vi "LDC501Control.vi"() -> ()   [LabVIEW 2021]
uses:
  <vilib>/Utility/file.llb/Write Delimited Spreadsheet (DBL).vi
panel:
  in  "LASER CONFIGURATION 2":T1={"LD Range"=1, "Laser Control Mode"=0, "Laser Mod On/OFF"=1, "Laser Mod BW"=1} {"Laser Mod BW" items=["Low", "High"]; "Laser Mod On/OFF" items=["OFF", "ON"]; "Laser Control Mode" items=["CC", "CP"]; "LD Range" items=["250mA", "500mA"]}
  in  "LASER CONFIGURATION":T1={"LD Range"=1, "Laser Control Mode"=0, "Laser Mod On/OFF"=1, "Laser Mod BW"=1} {"Laser Mod BW" items=["Low", "High"]; "Laser Mod On/OFF" items=["OFF", "ON"]; "Laser Control Mode" items=["CC", "CP"]; "LD Range" items=["250mA", "500mA"]}
  in  "LASER LIMIT & TRIP-OFF 2":T2
  in  "LASER LIMIT & TRIP-OFF":T2
  out "Laser On 2":bool
  out "LD Voltage":dbl
  out "LD Current":dbl
  in  "Laser ON/OFF 2":bool
  in  "LD Setting Point":dbl
  in  "Repump Laser":refnum<visa-resource-name>="LDC_Repump"
  out "error out 2":errorcluster
  out "error out":errorcluster
  out "LD Voltage":dbl
  out "LD Current":dbl
  in  "LD Setting Point":dbl
  out "Laser On":bool
  in  "Laser ON/OFF":bool
  in  "Refresh Monitor":bool
  in  "Trap Laser":refnum<visa-resource-name>="LDC_Trap"
  in  "Stop":bool
  in  "Export Setting":bool
  in  "Import Setting":bool
  # "Trap & Repump Laser Controller"
  # "LD Currernt Range"
  # "Laser Control Mode"
  # "Laser Mod On/OFF"
  # "Laser Mod BW"
  # "LD Currernt Range"
  # "Laser Control Mode"
  # "Laser Mod On/OFF"
  # "Laser Mod BW"
  # "Laser Trip-off on"
  # "Current Limit"
  # "TEC Off"
  # "Min Temperature"
  # "Max Temperature"
  # "Laser Trip-off on"
  # "Current Limit"
  # "TEC Off"
  # "Min Temperature"
  # "Max Temperature"
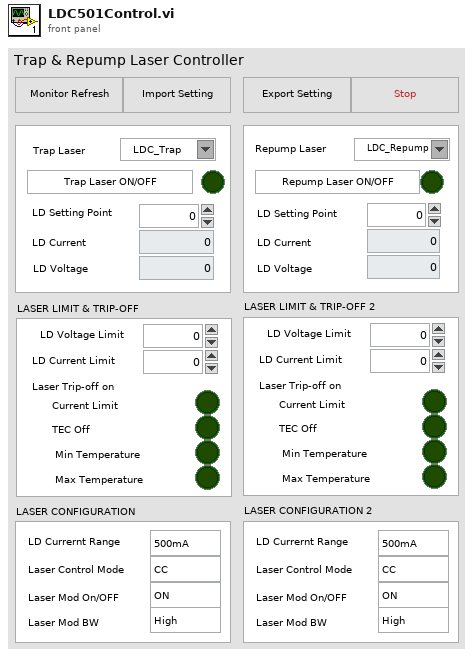
[diagram p1: front panel]
types:
  T1 = cluster{"LD Range":u16, "Laser Control Mode":u16, "Laser Mod On/OFF":u16, "Laser Mod BW":u16}
  T2 = cluster{"LD Voltage Limit":dbl, "LD Current Limit":dbl, "Laser Trip-off on Current Limit":bool, "Laser Trip-off on TEC Off":bool, "Laser Trip-off on Min Temperature":bool, "Laser Trip-off on Max Temperature":bool}
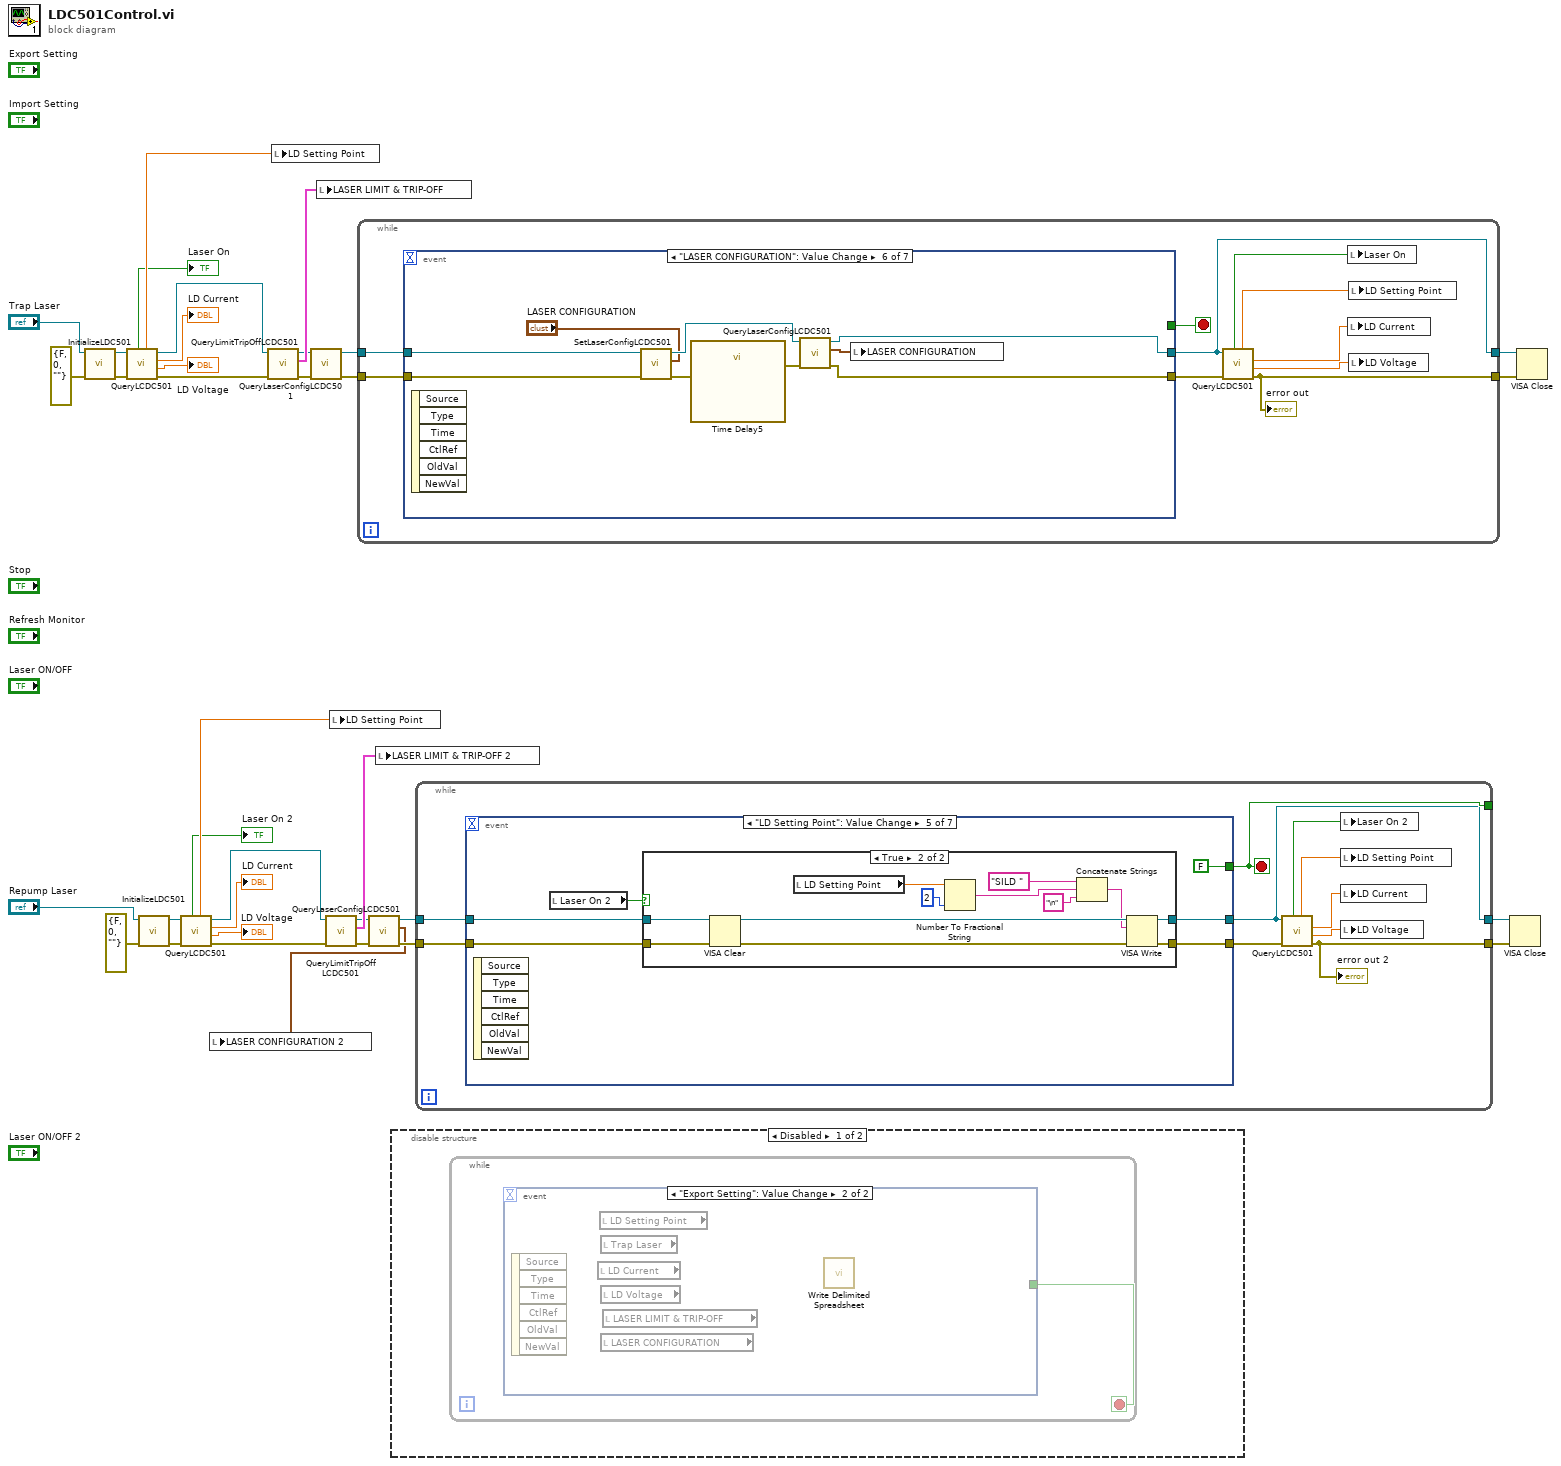
[diagram p0: block diagram]
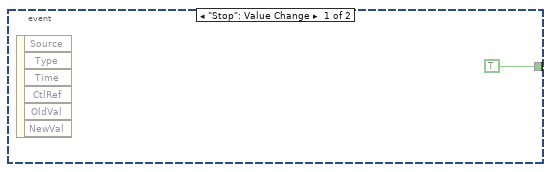
[diagram p2: hidden frame]
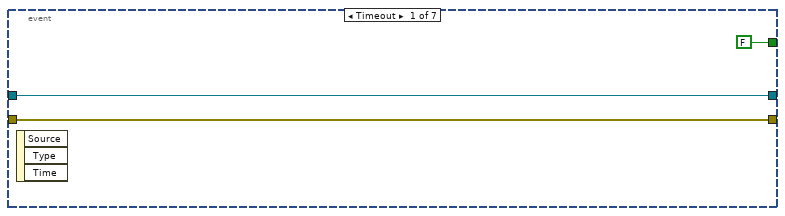
[diagram p4: hidden frame]
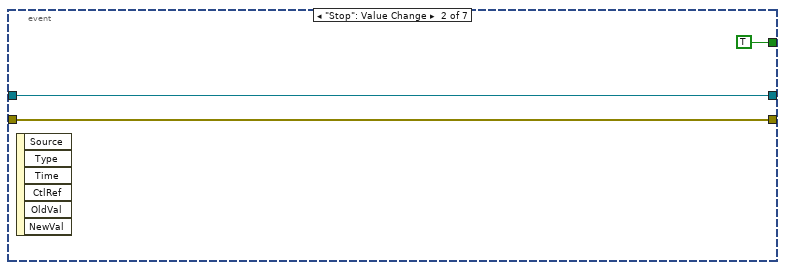
[diagram p5: hidden frame]
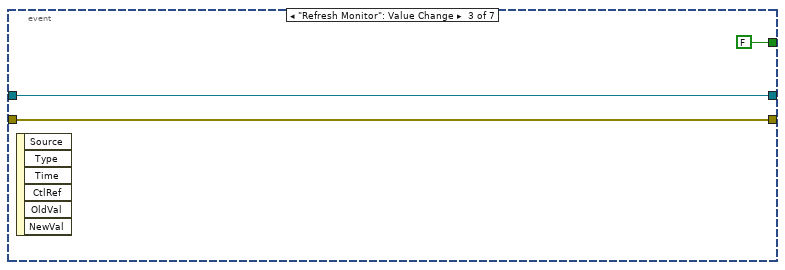
[diagram p6: hidden frame]
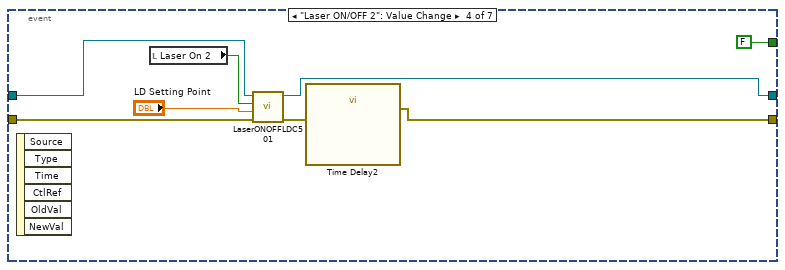
[diagram p7: hidden frame]
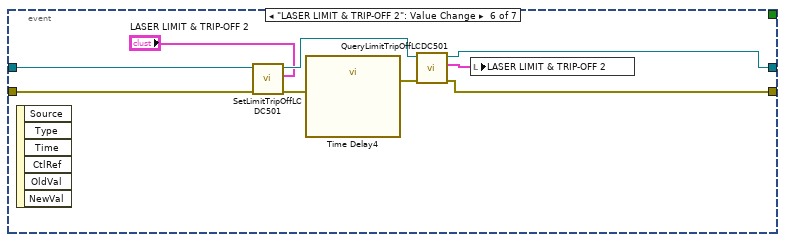
[diagram p9: hidden frame]
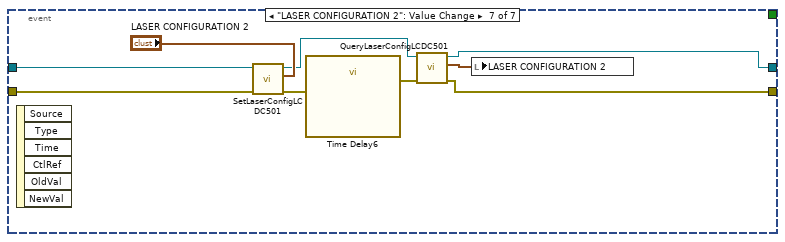
[diagram p10: hidden frame]
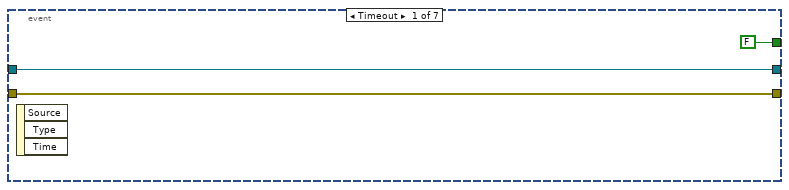
[diagram p11: hidden frame]
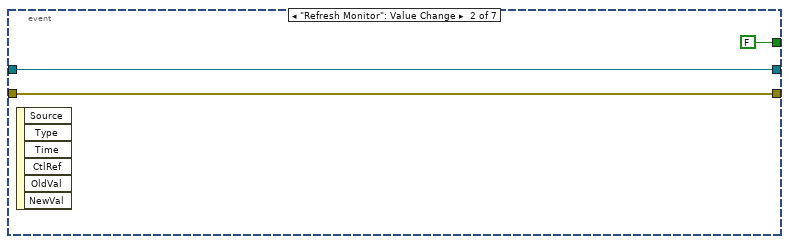
[diagram p12: hidden frame]
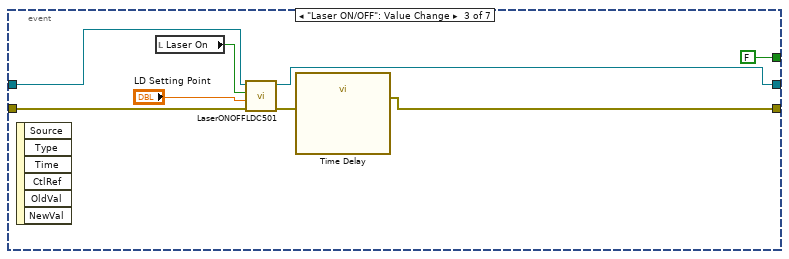
[diagram p13: hidden frame]
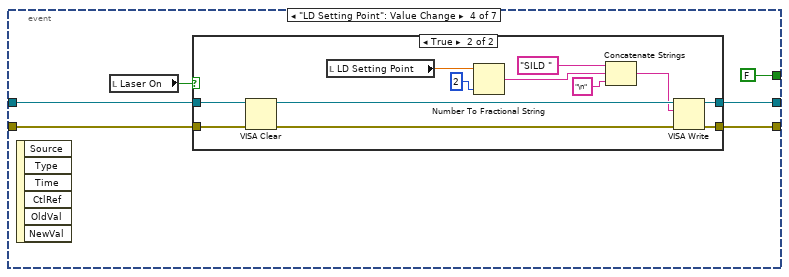
[diagram p14: hidden frame]
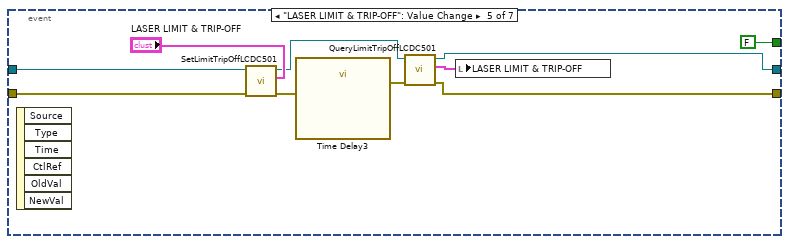
[diagram p16: hidden frame]
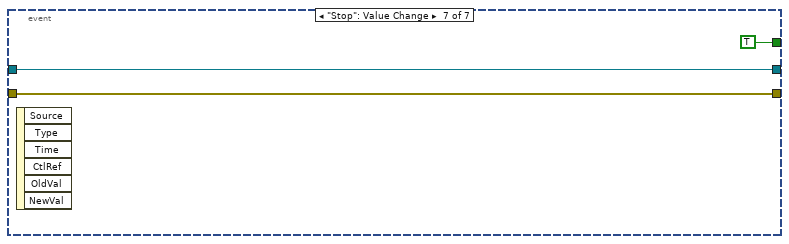
[diagram p17: hidden frame]
diagram:
  n1 = call "InitializeLDC501.vi"("error in (no error)"=errorcluster {"status"=FALSE, "code"=0, "source"=""}, "VISA resource name"="Trap Laser") -> ("error out"=w33:errorcluster, "VISA resource name out"=w32:refnum<visa-resource-name>)  [unwired: 8 in]
  n2 = call "QueryLCDC501.vi"("error in (no error)"=w33, "VISA resource name"=w32) -> ("error out"=w14:errorcluster, "LD Voltage"=→"LD Voltage":dbl, "LD Current"=→"LD Current":dbl, "VISA resource name out"=w15:refnum<visa-resource-name>, "LD Setting Point"=w29:dbl, "Laser status"=→"Laser On":bool)  [unwired: 4 in]
  n3 = call "InitializeLDC501.vi"("error in (no error)"=errorcluster {"status"=FALSE, "code"=0, "source"=""}, "VISA resource name"="Repump Laser") -> ("error out"=w25:errorcluster, "VISA resource name out"=w24:refnum<visa-resource-name>)  [unwired: 8 in]
  n4 = call "QueryLCDC501.vi"("error in (no error)"=w25, "VISA resource name"=w24) -> ("error out"=w12:errorcluster, "LD Voltage"=→"LD Voltage":dbl, "LD Current"=→"LD Current":dbl, "VISA resource name out"=w11:refnum<visa-resource-name>, "LD Setting Point"=w21:dbl, "Laser status"=→"Laser On 2":bool)  [unwired: 4 in]
  n5 = call "QueryLimitTripOffLCDC501.vi"("error in (no error)"=w14, "VISA resource name"=w15) -> ("error out"=w8:errorcluster, "LASER LIMIT & TRIP-OFF"=w13:T2, "VISA resource name out"=w9:refnum<visa-resource-name>)  [unwired: 7 in]
  n6 = local write "LD Setting Point"(w29) -> ()
  n7 = call "QueryLaserConfigLCDC501.vi"("error in (no error)"=w8, "VISA resource name"=w9) -> ("error out"=w6:errorcluster, "VISA resource name out"=w7:refnum<visa-resource-name>)  [unwired: 7 in, 1 out]
  n8 = local write "LASER LIMIT & TRIP-OFF"(w13) -> ()
  n9 = call "QueryLimitTripOffLCDC501.vi"("error in (no error)"=w12, "VISA resource name"=w11) -> ("error out"=w4:errorcluster, "LASER LIMIT & TRIP-OFF"=w10:T2, "VISA resource name out"=w5:refnum<visa-resource-name>)  [unwired: 7 in]
  n10 = local write "LD Setting Point"(w21) -> ()
  n11 = while {
    tunnel: w7 -> [w45]
    tunnel: w6 -> [w44]
    tunnel: [w37] -> w19
    tunnel: [w36] -> w18
    stop <- w38 stop-if-true
    n12 = event shown="[5] \"LASER CONFIGURATION\": Value Change" {
      selector: _ -> [_ _ _ _ _ _ _]
      dyn-events: _ -> [_ _ _ _ _ _ _]
      timeout: _ -> [_ _ _ _ _ _ _]
      tunnel: w45 -> [w47 w51 w59 w64 w89 w98 w101]
      tunnel: w44 -> [w46 w50 w58 w63 w88 w97 w100]
      tunnel: [w46 w50 w53 w62 w83 w90 w100] -> w43
      tunnel: [w47 w51 w56 w61 w84 w91 w101] -> w36
      tunnel: [FALSE FALSE FALSE FALSE FALSE _ TRUE] -> w38
      event Timeout {
        n13 = event-data() -> ()  [unwired: 1 in, 3 out]
      }
      event "Refresh Monitor": Value Change {
        n14 = event-data() -> ()  [unwired: 1 in, 6 out]
      }
      event "Laser ON/OFF": Value Change {
        n15 = event-data() -> ()  [unwired: 1 in, 6 out]
        n16 = local read "Laser On"() -> (w57:bool)
        n17 = call "LaserONOFFLDC501.vi"("error in (no error)"=w58, "LD Setting Point (If ON)"="LD Setting Point", "Currnet ON/OFF"=w57, "VISA resource name"=w59) -> ("error out"=w54:errorcluster, "VISA resource name out"=w56:refnum<visa-resource-name>)  [unwired: 6 in]
        n18 = call "Time Delay"("error in (no error)"=w54) -> ("error out"=w53:errorcluster)  [unwired: 10 in]
      }
      event "LD Setting Point": Value Change {
        n19 = event-data() -> ()  [unwired: 1 in, 6 out]
        n20 = local read "Laser On"() -> (w65:bool)
        n21 = case shown="True" w65 {
          tunnel: w64 -> [w67 w71]
          tunnel: w63 -> [w66 w70]
          tunnel: [w66 w69] -> w62
          tunnel: [w67 w68] -> w61
          frame False {
          }
          frame True {
            n22 = VISA Clear(VISA resource name=w71, error in (no error)=w70) -> (VISA resource name out=w78:refnum<visa-resource-name>, error out=w79:errorcluster)
            n23 = local read "LD Setting Point"() -> (w72:dbl)
            n24 = Number To Fractional String(number=w72, precision (6)=i16 2) -> (F-format string=w76:string)  [unwired: 2 in]
            n25 = Concatenate Strings("SILD " ("write buffer"), w76, "\n" ("write buffer")) -> (w77:string)
            n26 = VISA Write(VISA resource name=w78, write buffer=w77, error in (no error)=w79) -> (VISA resource name out=w68:refnum<visa-resource-name>, error out=w69:errorcluster)  [unwired: 1 out]
          }
        }
      }
      event "LASER LIMIT & TRIP-OFF": Value Change {
        n27 = event-data() -> ()  [unwired: 1 in, 6 out]
        n28 = call "SetLimitTripOffLCDC501.vi"("LASER LIMIT & TRIP-OFF"="LASER LIMIT & TRIP-OFF", "error in (no error)"=w88, "VISA resource name"=w89) -> ("error out"=w81:errorcluster, "VISA resource name out"=w86:refnum<visa-resource-name>)  [unwired: 7 in]
        n29 = call "Time Delay3"("error in (no error)"=w81) -> ("error out"=w80:errorcluster)  [unwired: 10 in]
        n30 = call "QueryLimitTripOffLCDC501.vi"("error in (no error)"=w80, "VISA resource name"=w86) -> ("error out"=w83:errorcluster, "LASER LIMIT & TRIP-OFF"=w85:T2, "VISA resource name out"=w84:refnum<visa-resource-name>)  [unwired: 7 in]
        n31 = local write "LASER LIMIT & TRIP-OFF"(w85) -> ()
      }
      event "LASER CONFIGURATION": Value Change {
        n32 = event-data() -> ()  [unwired: 1 in, 6 out]
        n33 = call "SetLaserConfigLCDC501.vi"("LASER CONFIGURATION"="LASER CONFIGURATION", "error in (no error)"=w97, "VISA resource name"=w98) -> ("error out"=w96:errorcluster, "VISA resource name out"=w94:refnum<visa-resource-name>)  [unwired: 7 in]
        n34 = call "Time Delay5"("error in (no error)"=w96) -> ("error out"=w95:errorcluster)  [unwired: 10 in]
        n35 = call "QueryLaserConfigLCDC501.vi"("error in (no error)"=w95, "VISA resource name"=w94) -> ("error out"=w90:errorcluster, "LASER CONFIGURATION"=w92:T1, "VISA resource name out"=w91:refnum<visa-resource-name>)  [unwired: 7 in]
        n36 = local write "LASER CONFIGURATION"(w92) -> ()
      }
      event "Stop": Value Change {
        n37 = event-data() -> ()  [unwired: 1 in, 6 out]
      }
    }
    n38 = call "QueryLCDC501.vi"("error in (no error)"=w43, "VISA resource name"=w36) -> ("error out"=w37:errorcluster, "LD Voltage"=w42:dbl, "LD Current"=w41:dbl, "LD Setting Point"=w39:dbl, "Laser status"=w40:bool)  [unwired: 4 in, 1 out]
    "error out" <- w37
    n39 = local write "Laser On"(w40) -> ()
    n40 = local write "LD Current"(w41) -> ()
    n41 = local write "LD Setting Point"(w39) -> ()
    n42 = local write "LD Voltage"(w42) -> ()
  }
  n43 = call "QueryLaserConfigLCDC501.vi"("error in (no error)"=w4, "VISA resource name"=w5) -> ("error out"=w3:errorcluster, "LASER CONFIGURATION"=w1:T1, "VISA resource name out"=w2:refnum<visa-resource-name>)  [unwired: 7 in]
  n44 = local write "LASER CONFIGURATION 2"(w1) -> ()
  n45 = local write "LASER LIMIT & TRIP-OFF 2"(w10) -> ()
  n46 = disable-structure shown="Disabled" {
    frame Disabled {
      n47 = while {
        stop <- w102 stop-if-true
        n48 = event shown="[1] \"Export Setting\": Value Change" {
          selector: _ -> [_ _]
          dyn-events: _ -> [_ _]
          timeout: _ -> [_ _]
          tunnel: [TRUE _] -> w102
          event "Stop": Value Change {
            n49 = event-data() -> ()  [unwired: 1 in, 6 out]
          }
          event "Export Setting": Value Change {
            n50 = event-data() -> ()  [unwired: 1 in, 6 out]
            n51 = local read "LD Current"() -> ()  [unwired: 1 out]
            n52 = local read "LD Setting Point"() -> ()  [unwired: 1 out]
            n53 = local read "Trap Laser"() -> ()  [unwired: 1 out]
            n54 = local read "LD Voltage"() -> ()  [unwired: 1 out]
            n55 = local read "LASER CONFIGURATION"() -> ()  [unwired: 1 out]
            n56 = local read "LASER LIMIT & TRIP-OFF"() -> ()  [unwired: 1 out]
            n57 = call-poly <vilib>:"Write Delimited Spreadsheet.vi"() -> ()  [unwired: 14 in, 2 out]
          }
        }
      }
    }
    frame Enabled {
    }
  }
  n58 = while {
    tunnel: w2 -> [w113]
    tunnel: w3 -> [w112]
    tunnel: [w106] -> _
    tunnel: [w105] -> w17
    tunnel: [w104] -> w16
    stop <- w106 stop-if-true
    n59 = event shown="[4] \"LD Setting Point\": Value Change" {
      selector: _ -> [_ _ _ _ _ _ _]
      dyn-events: _ -> [_ _ _ _ _ _ _]
      timeout: _ -> [_ _ _ _ _ _ _]
      tunnel: w113 -> [w115 w119 w122 w130 w135 w156 w166]
      tunnel: w112 -> [w114 w118 w121 w129 w134 w155 w165]
      tunnel: [w114 w118 w121 w124 w133 w154 w161] -> w111
      tunnel: [w115 w119 w122 w127 w132 w153 w162] -> w104
      tunnel: [FALSE ("Stop") TRUE ("Stop") FALSE ("Stop") FALSE ("Stop") FALSE ("Stop") _ _] -> w106
      event Timeout {
        n60 = event-data() -> ()  [unwired: 1 in, 3 out]
      }
      event "Stop": Value Change {
        n61 = event-data() -> ()  [unwired: 1 in, 6 out]
      }
      event "Refresh Monitor": Value Change {
        n62 = event-data() -> ()  [unwired: 1 in, 6 out]
      }
      event "Laser ON/OFF 2": Value Change {
        n63 = event-data() -> ()  [unwired: 1 in, 6 out]
        n64 = local read "Laser On 2"() -> (w128:bool)
        n65 = call "LaserONOFFLDC501.vi"("error in (no error)"=w129, "LD Setting Point (If ON)"="LD Setting Point", "Currnet ON/OFF"=w128, "VISA resource name"=w130) -> ("error out"=w125:errorcluster, "VISA resource name out"=w127:refnum<visa-resource-name>)  [unwired: 6 in]
        n66 = call "Time Delay2"("error in (no error)"=w125) -> ("error out"=w124:errorcluster)  [unwired: 10 in]
      }
      event "LD Setting Point": Value Change {
        n67 = event-data() -> ()  [unwired: 1 in, 6 out]
        n68 = local read "Laser On 2"() -> (w136:bool)
        n69 = case shown="True" w136 {
          tunnel: w135 -> [w138 w142]
          tunnel: w134 -> [w137 w141]
          tunnel: [w137 w140] -> w133
          tunnel: [w138 w139] -> w132
          frame False {
          }
          frame True {
            n70 = VISA Clear(VISA resource name=w142, error in (no error)=w141) -> (VISA resource name out=w149:refnum<visa-resource-name>, error out=w150:errorcluster)
            n71 = local read "LD Setting Point"() -> (w143:dbl)
            n72 = Number To Fractional String(number=w143, precision (6)=i16 2) -> (F-format string=w147:string)  [unwired: 2 in]
            n73 = Concatenate Strings("SILD " ("write buffer"), w147, "\n" ("write buffer")) -> (w148:string)
            n74 = VISA Write(VISA resource name=w149, write buffer=w148, error in (no error)=w150) -> (VISA resource name out=w139:refnum<visa-resource-name>, error out=w140:errorcluster)  [unwired: 1 out]
          }
        }
      }
      event "LASER LIMIT & TRIP-OFF 2": Value Change {
        n75 = event-data() -> ()  [unwired: 1 in, 6 out]
        n76 = call "SetLimitTripOffLCDC501.vi"("LASER LIMIT & TRIP-OFF"="LASER LIMIT & TRIP-OFF 2", "error in (no error)"=w155, "VISA resource name"=w156) -> ("error out"=w158:errorcluster, "VISA resource name out"=w159:refnum<visa-resource-name>)  [unwired: 7 in]
        n77 = call "Time Delay4"("error in (no error)"=w158) -> ("error out"=w157:errorcluster)  [unwired: 10 in]
        n78 = call "QueryLimitTripOffLCDC501.vi"("error in (no error)"=w157, "VISA resource name"=w159) -> ("error out"=w154:errorcluster, "LASER LIMIT & TRIP-OFF"=w151:T2, "VISA resource name out"=w153:refnum<visa-resource-name>)  [unwired: 7 in]
        n79 = local write "LASER LIMIT & TRIP-OFF 2"(w151) -> ()
      }
      event "LASER CONFIGURATION 2": Value Change {
        n80 = event-data() -> ()  [unwired: 1 in, 6 out]
        n81 = call "SetLaserConfigLCDC501.vi"("LASER CONFIGURATION"="LASER CONFIGURATION 2", "error in (no error)"=w165, "VISA resource name"=w166) -> ("error out"=w168:errorcluster, "VISA resource name out"=w163:refnum<visa-resource-name>)  [unwired: 7 in]
        n82 = call "Time Delay6"("error in (no error)"=w168) -> ("error out"=w167:errorcluster)  [unwired: 10 in]
        n83 = call "QueryLaserConfigLCDC501.vi"("error in (no error)"=w167, "VISA resource name"=w163) -> ("error out"=w161:errorcluster, "LASER CONFIGURATION"=w160:T1, "VISA resource name out"=w162:refnum<visa-resource-name>)  [unwired: 7 in]
        n84 = local write "LASER CONFIGURATION 2"(w160) -> ()
      }
    }
    n85 = call "QueryLCDC501.vi"("error in (no error)"=w111, "VISA resource name"=w104) -> ("error out"=w105:errorcluster, "LD Voltage"=w110:dbl, "LD Current"=w109:dbl, "LD Setting Point"=w107:dbl, "Laser status"=w108:bool)  [unwired: 4 in, 1 out]
    "error out 2" <- w105
    n86 = local write "Laser On 2"(w108) -> ()
    n87 = local write "LD Setting Point"(w107) -> ()
    n88 = local write "LD Current"(w109) -> ()
    n89 = local write "LD Voltage"(w110) -> ()
  }
  n90 = VISA Close(VISA resource name=w16, error in (no error)=w17) -> ()  [unwired: 1 out]
  n91 = VISA Close(VISA resource name=w18, error in (no error)=w19) -> ()  [unwired: 1 out]
